vi "Logarithm Fit Coefficients.vi"(0 "Y":dbl[](array[numeric]), 1 "base":dbl(ring)=2.71828 items=["e"=2.71828, "2"=2.0, "10"=10.0], 5 "X":dbl[](array[numeric]), 7 "Weight":dbl[](array[numeric]), 9 "tolerance":dbl=0.0001, 11 "method":T1 items=["Least Square", "Least Absolute Residual", "Bisquare"]) -> (4 "amplitude":dbl, 6 "scale":dbl, 15 "error":i32)   [LabVIEW 2014, in "NI_AALPro.lvlib"]
doc: "Returns the <B>amplitude</B> and <B>scale</B> of the logarithmic fit for a data set (<B>X</B>, <B>Y</B>)."
uses:
  NI_AALPro.lvlib
  Curve Fitting Criteria.ctl
panel:
  # "Logarithm Fit Coefficients"
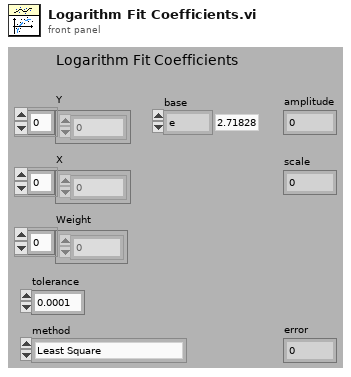
[diagram p1: front panel]
types:
  T1 = typedef "NI_AALPro.lvlib/Curve Fitting Criteria.ctl" = u16
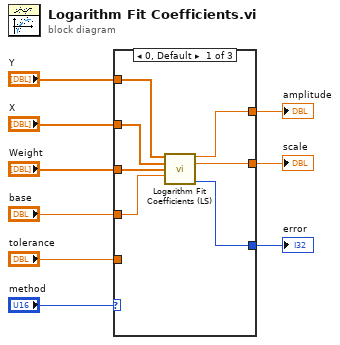
[diagram p0: block diagram]
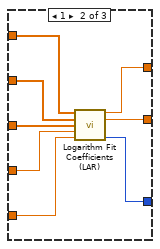
[diagram p2: hidden frame]
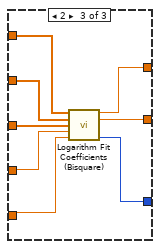
[diagram p3: hidden frame]
diagram:
  n1 = case shown="0, Default" "method" {
    tunnel: "Y" -> [w16 w24 w32]
    tunnel: "X" -> [w15 w23 w31]
    tunnel: "Weight" -> [w14 w22 w30]
    tunnel: "base" -> [w13 w21 w29]
    tunnel: [w12 w18 w26] -> w4
    tunnel: [w11 w19 w27] -> w3
    tunnel: [w10 w17 w25] -> w2
    tunnel: "tolerance" -> [_ w20 w28]
    frame 0, Default {
      n2 = call "Logarithm Fit Coefficients (LS).vi"("Y"=w16, "X"=w15, "Weight"=w14, "base of logarithm"=w13) -> ("amplitude"=w11:dbl, "scale"=w12:dbl, "error"=w10:i32)  [unwired: 9 out]
    }
    frame 1 {
      n3 = call "Logarithm Fit Coefficients (LAR).vi"("Y"=w24, "X"=w23, "Weight"=w22, "base of logarithm"=w21, "tol"=w20) -> ("amplitude"=w19:dbl, "scale"=w18:dbl, "error"=w17:i32)  [unwired: 8 out]
    }
    frame 2 {
      n4 = call "Logarithm Fit Coefficients (Bisquare).vi"("Y"=w32, "X"=w31, "Weight"=w30, "base of logarithm"=w29, "tol"=w28) -> ("amplitude"=w27:dbl, "scale"=w26:dbl, "error"=w25:i32)  [unwired: 8 out]
    }
  }
  "amplitude" <- w3
  "scale" <- w4
  "error" <- w2
